vi "SSC Digital Write Source Waveform [Broadcast].vi"(0 "Digital SSC in":T1[](array[typedef]), 1 "Waveform Name":string, 5 "Waveform Data":u32[](array[numeric]) format="%.0x", 7 "Expand to Minimum Size?":bool caption="Expand to Minimum Size? (F)", 9 "Minimum Size":i32=128 caption="Minimum Size (128)", 11 "error in":errorcluster) -> (4 "Digital SSC out":T1[](array[typedef]), 15 "error out":errorcluster)   [LabVIEW 2019]
doc: "Writes the same waveform data to all sites connected to the specified pin(s) and pin group(s). Use this instance of the niDigital Write Source Waveform VI if you set the data mapping parameter of your source waveform to Broadcast."
uses:
  SSC Digital.ctl
  <instrlib>/niDigital/niDigital.llb/niDigital Write Source Waveform (Broadcast U32).vi
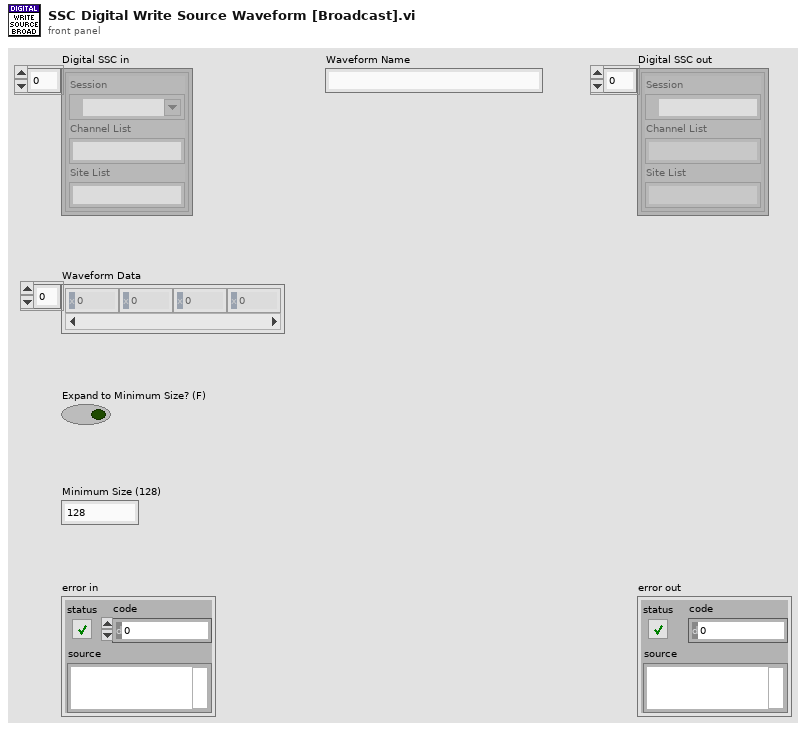
[diagram p1: front panel]
types:
  T1 = typedef "SSC Digital.ctl" = cluster{"Session":refnum<k15>, "Channel List":string, "Site List":string}
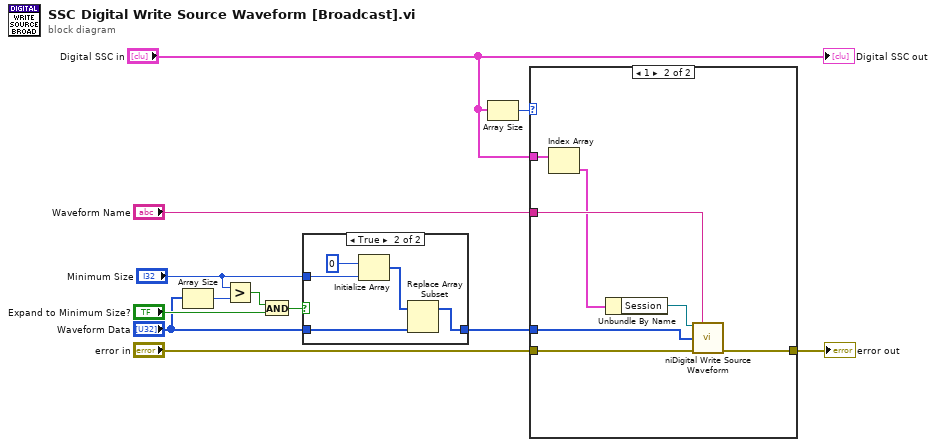
[diagram p0: block diagram]
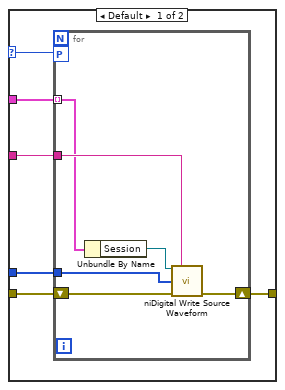
[diagram p2: hidden frame]
diagram:
  n1 = Array Size(array="Waveform Data") -> (size(s)=w11:i32)
  n2 = Greater?(x="Minimum Size", y=w11) -> (0:w8:bool)
  n3 = And(x=w8, y="Expand to Minimum Size?") -> (x .and. y?=w9:bool)
  n4 = case shown="True" w9 {
    tunnel: "Waveform Data" -> [w13 w16]
    tunnel: [w13 w15] -> w6
    tunnel: "Minimum Size" -> [_ w14]
    frame False {
    }
    frame True {
      n5 = Initialize Array(u32 0 ("Numeric"), w14) -> (w17:u32[])
      n6 = Replace Array Subset(array=w17, new element=w16) -> (w15:u32[])  [unwired: 1 in]
    }
  }
  n7 = Array Size(array="Digital SSC in") -> (size(s)=w1:i32)
  n8 = case shown="1" w1 {
    selector: w1 -> [w19 _]
    tunnel: "Waveform Name" -> [w24 w37]
    tunnel: w6 -> [w23 w36]
    tunnel: "error in" -> [w22 w35]
    tunnel: [w21 w34] -> w3
    tunnel: "Digital SSC in" -> [w20 w33]
    frame Default {
      n9 = for {
        tunnel: w24 -> [w30]
        workers-P: w19 -> [_]
        tunnel: w23 -> [w27]
        tunnel: w20 -> [w26] mode=indexing
        shift-right: [w28] -> w21
        shift-left: w22 -> [w29]
        n10 = Unbundle By Name(w26) -> ("Session"=w25:refnum<k15>)
        n11 = call-poly <instrlib>:"niDigital Write Source Waveform.vi"("instrument handle"=w25, "waveform name"=w30, "waveform data"=w27, "error in"=w29) -> ("error out"=w28:errorcluster)  [unwired: 10 in, 1 out]
      }
    }
    frame 1 {
      n12 = Index Array(array=w33) -> (element=w31:T1)  [unwired: 1 in]
      n13 = Unbundle By Name(w31) -> ("Session"=w32:refnum<k15>)
      n14 = call-poly <instrlib>:"niDigital Write Source Waveform.vi"("instrument handle"=w32, "waveform name"=w37, "waveform data"=w36, "error in"=w35) -> ("error out"=w34:errorcluster)  [unwired: 10 in, 1 out]
    }
  }
  "error out" <- w3
  "Digital SSC out" <- "Digital SSC in"
